vi "DoubleSolenoidPulse-test.vi"() -> ()   [LabVIEW 2019]
uses:
  <vilib>/Rock Robotics/WPI/ThirdParty/JAS_Junk/TrajLib/Trajectory_Library.lvlib
  <vilib>/Rock Robotics/WPI/Solenoid/WPI_SolenoidValue.ctl
panel:
  out "Solenoid Cmd":T1
  in  "Solenoid Pulse\nTime\nSeconds":dbl=1.0 format="%#_13g"
  in  "Robot Enabled":bool
  in  "Demand":bool
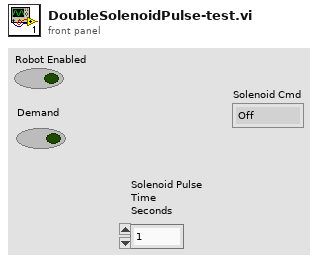
[diagram p1: front panel]
types:
  T1 = typedef "WPI_SolenoidValue.ctl" = enum16{"Off", "On", "Forward", "Reverse"}
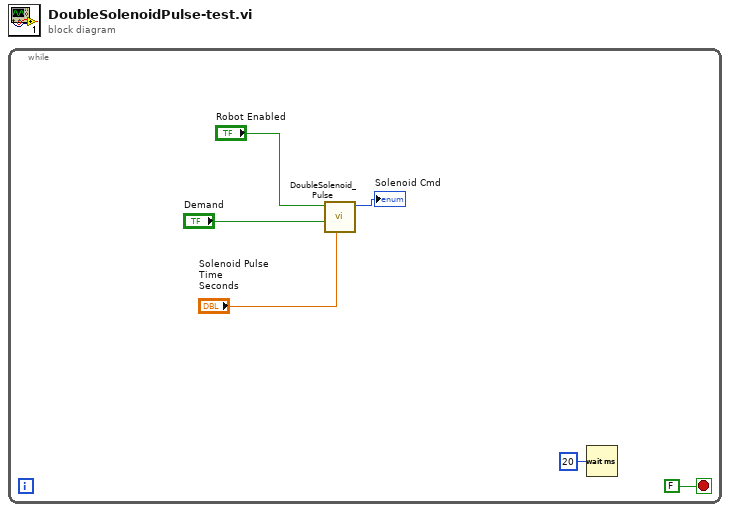
[diagram p0: block diagram]
diagram:
  n1 = while {
    stop <- FALSE stop-if-true
    n2 = call <vilib>:"DoubleSolenoid_Pulse.vi"("Solenoid Pulse\nTime\nSeconds"="Solenoid Pulse\nTime\nSeconds", "Solenoid Demand"="Demand", "Robot Enabled"="Robot Enabled") -> ("Solenoid Cmd"=→"Solenoid Cmd":T1)  [unwired: 8 in]
    n3 = Wait (ms)(milliseconds to wait=u32 20) -> ()  [unwired: 1 out]
  }
